vi "Detector_Controller_status_extract.vi"(10 "Status Headers":string, 11 "Status Controllers":string="\u0000Status of FitsHeader\n---------------------------------------------------------\r\nHeader0\r\nModify  : 20170204-171925568\r\nEXPTIMES: 1000\r\nEXPTIMEL: 1000\r\nNFRAMES : 1\r\nNGROUPS : 1\r\nOffsets : NOT loaded deu to write protection.\r\n          0x369 0x361 0x361 0x363 0x35a 0x357 0x360 0x361\r\n          0x34a 0x34c 0x347 0x349 0x34a 0x34b 0x349 0x349\r\n          0x351 0x350 0x353 0x351 0x351 0x351 0x350 0x353\r\n          0x350 0x352 0x353 0x352 0x353 0x351 0x351 0x355\r\n---------------------------------------------------------\r\nHeader1\r\nModify  : 20170204-171925571\r\nEXPTIMES: 2000\r\nEXPTIMEL: 1000\r\nNFRAMES : 1\r\nNGROUPS : 1\r\nOffsets : NOT loaded deu to write protection.\r\n          0x387 0x389 0x38a 0x389 0x388 0x38a 0x388 0x387\r\n          0x39c 0x39b 0x39d 0x39b 0x39d 0x39b 0x39c 0x39c\r\n          0x38f 0x38f 0x391 0x391 0x390 0x38e 0x38e 0x38e\r\n          0x38f 0x391 0x38e 0x390 0x38e 0x390 0x38f 0x38e\r\n---------------------------------------------------------") -> (2 "Params Det 1":i32[](array[numeric]), 3 "Params":i32[](array[numeric]))   [LabVIEW 2024]
uses:
  <vilib>/regexp/Match Regular Expression.xnode
panel:
  out "Controller status lines 2":string[](array[string])
  out "match + rest of string 4":string
  out "Status 2":bool[](array[boolean])
  out "Status":bool[](array[boolean])
  out "Controller status lines":string[](array[string])
  out "match + rest of string 3":string
  out "Satus of Detectors 1":string[](array[string])
  out "match + rest of string 2":string
  out "substring before match":string
  out "Array 2":i32[](array[numeric])
  out "Satus of Detector 0":string[](array[string])
  out "match + rest of string":string
  out "spreadsheet string":string
  out "after match":string
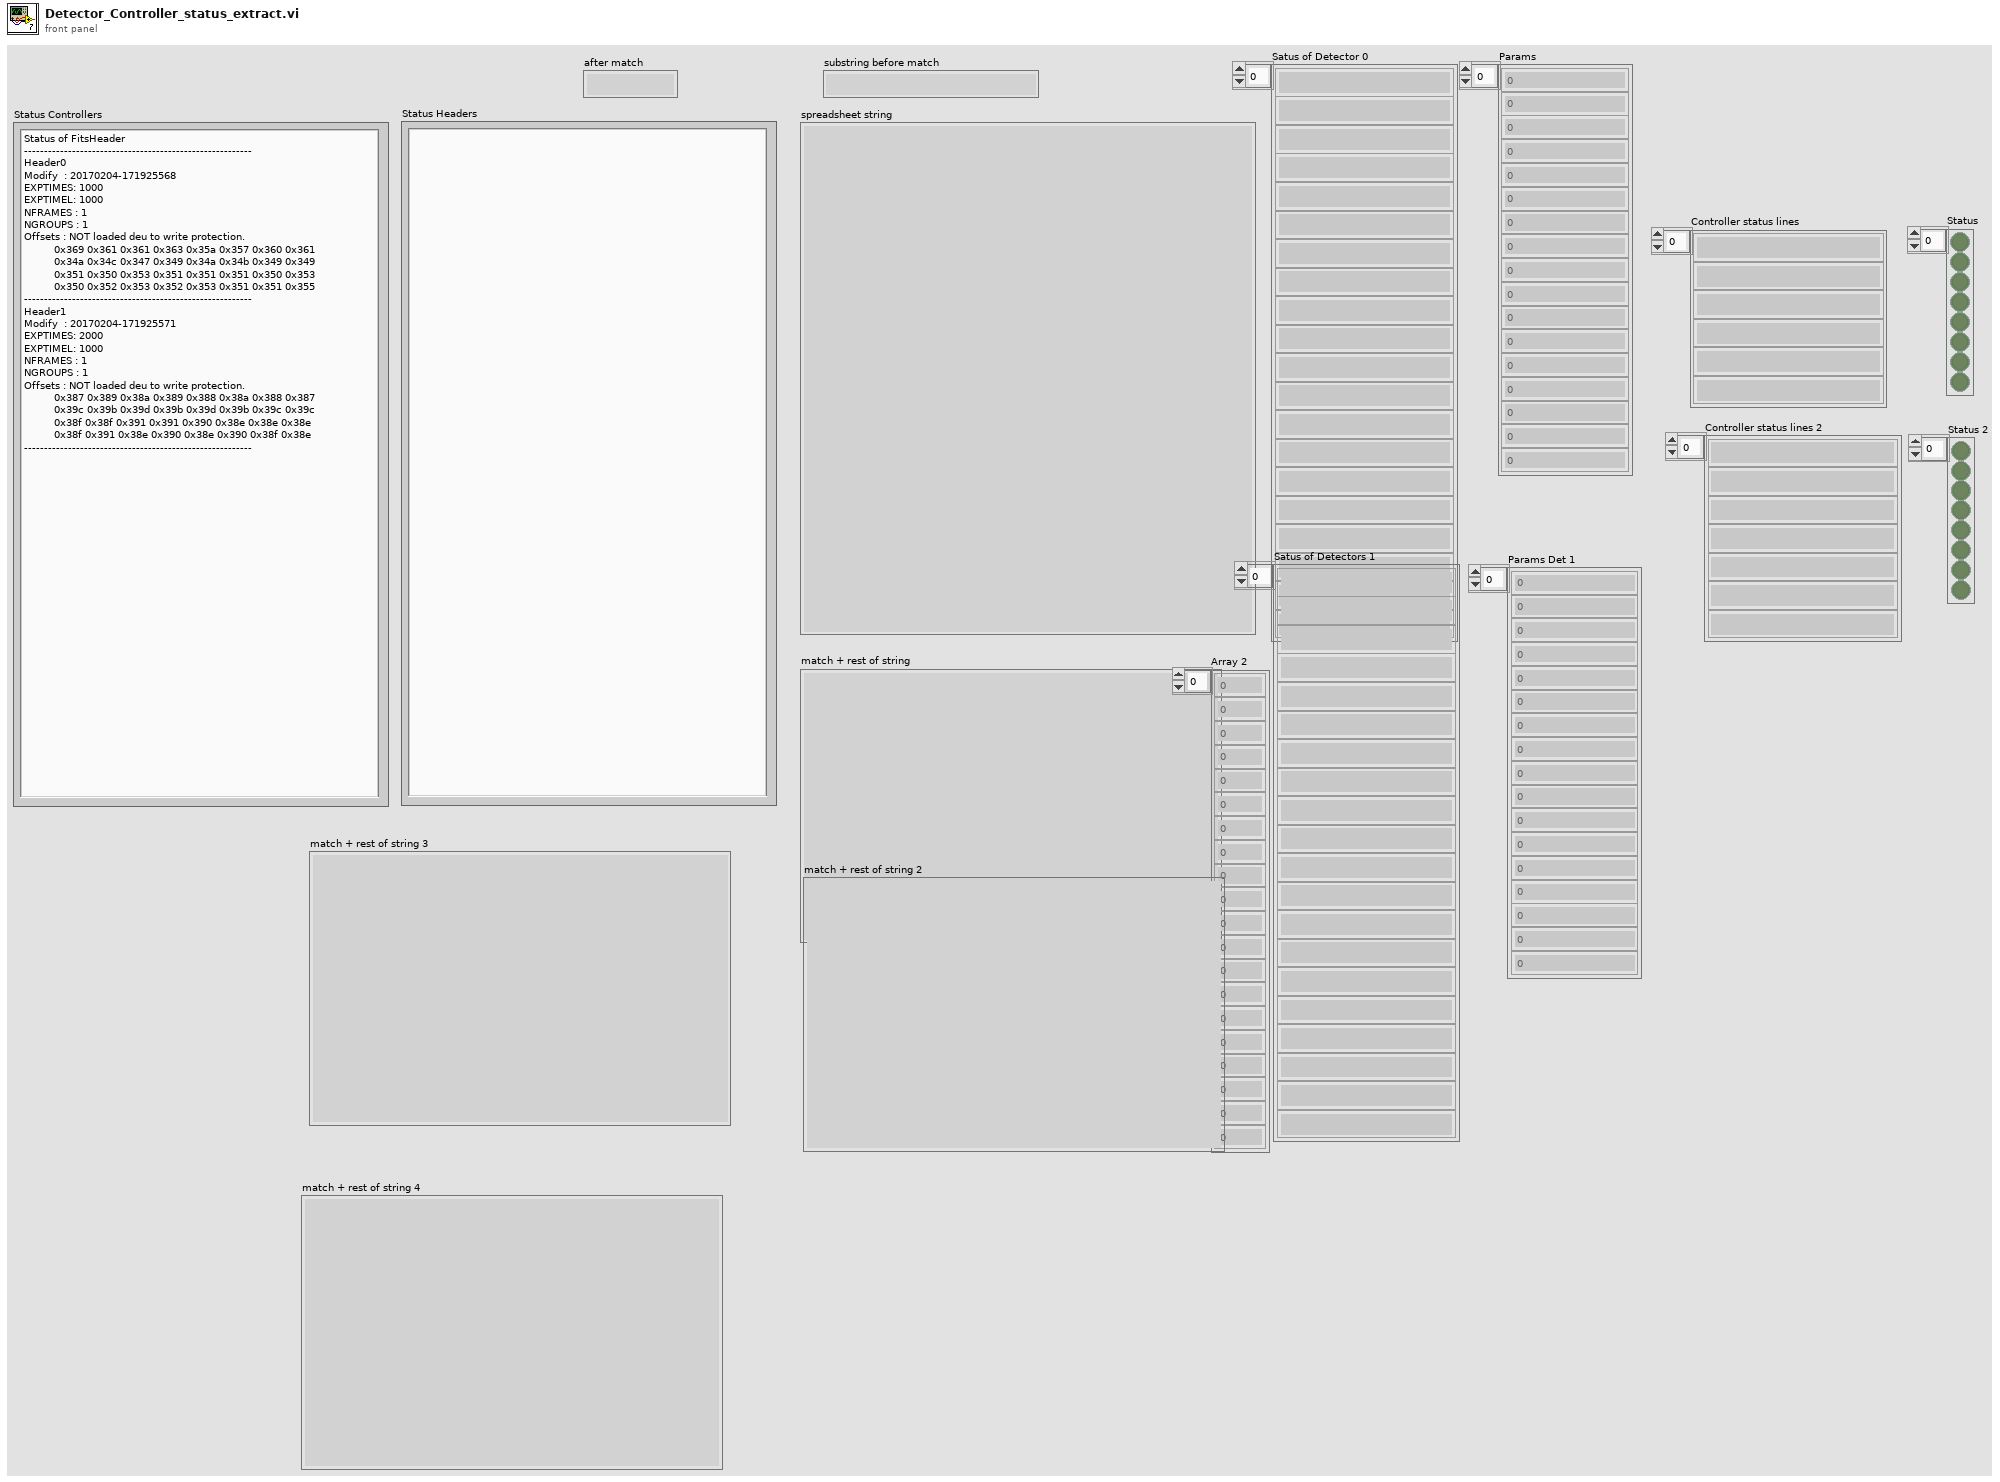
[diagram p1: front panel]
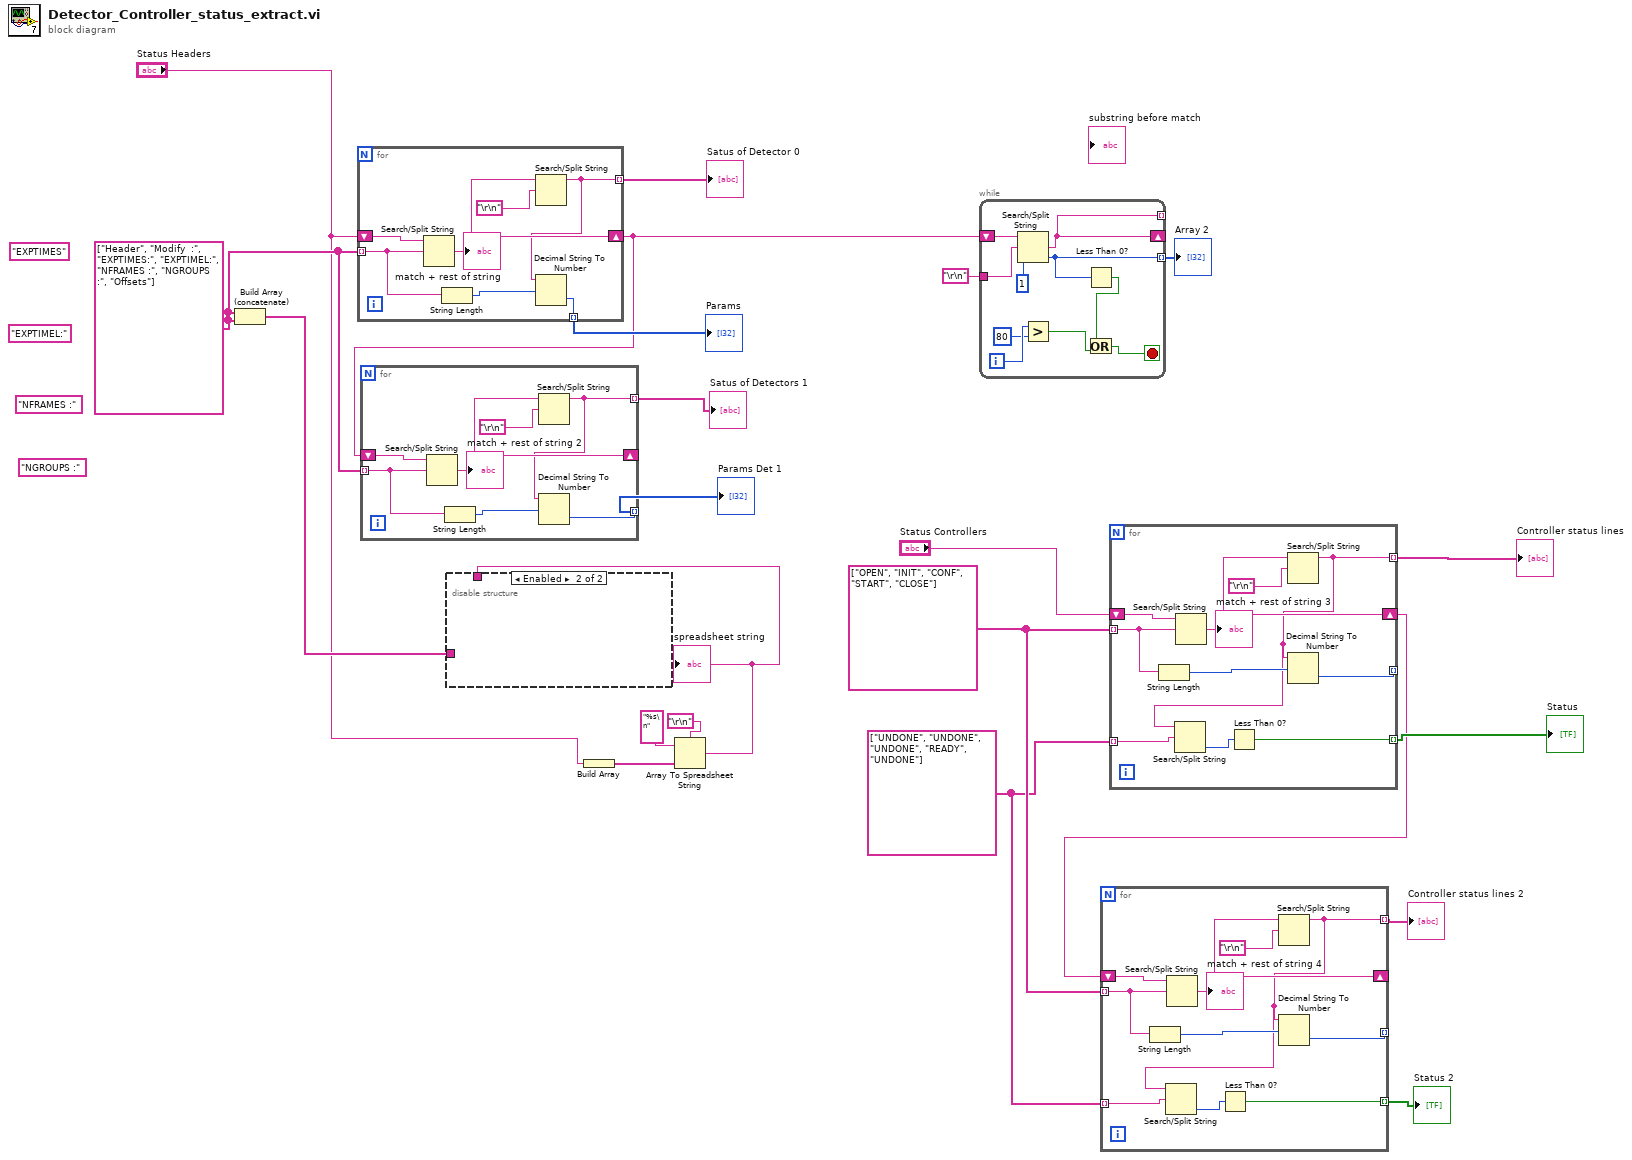
[diagram p0: block diagram]
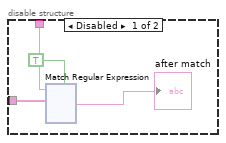
[diagram p2: hidden frame]
diagram:
  w3 = string[] ["UNDONE", "UNDONE", "UNDONE", "READY", "UNDONE"]
  w4 = string[] ["OPEN", "INIT", "CONF", "START", "CLOSE"]
  w12 = string[] ["Header", "Modify  :", "EXPTIMES:", "EXPTIMEL:", "NFRAMES :", "NGROUPS :", "Offsets"]
  (unwired) "NGROUPS :" ("Status Controllers")
  (unwired) "NFRAMES :" ("Status Controllers")
  (unwired) "EXPTIMEL:" ("Status Controllers")
  (unwired) "EXPTIMES" ("Status Controllers")
  n1 = Build Array (concatenate)(w12, w12) -> (w15:string[])
  n2 = for {
    tunnel: w12 -> [w24] mode=indexing
    tunnel: [w26] -> w16 mode=indexing
    shift-right: [w28] -> w13
    shift-left: "Status Headers" -> [w29]
    tunnel: [w25] -> w14 mode=indexing
    n3 = Search/Split String(string=w29, search string/char (-)=w24) -> (match + rest of string=w28:string)  [unwired: 1 in, 2 out]
    "match + rest of string" <- w28
    n4 = String Length(string=w24) -> (length=w23:i32)
    n5 = Search/Split String(string=w28, search string/char (-)="\r\n") -> (substring before match=w26:string)  [unwired: 1 in, 2 out]
    n6 = Decimal String To Number(string=w26, offset=w23) -> (number=w25:i32)  [unwired: 1 in, 1 out]
  }
  "Satus of Detector 0" <- w16
  "Params" <- w14
  n7 = for {
    tunnel: w12 -> [w31] mode=indexing
    tunnel: [w33] -> w11 mode=indexing
    shift-right: [w35] -> _
    shift-left: w13 -> [w36]
    tunnel: [w32] -> w10 mode=indexing
    n8 = Search/Split String(string=w36, search string/char (-)=w31) -> (match + rest of string=w35:string)  [unwired: 1 in, 2 out]
    "match + rest of string 2" <- w35
    n9 = String Length(string=w31) -> (length=w30:i32)
    n10 = Search/Split String(string=w35, search string/char (-)="\r\n") -> (substring before match=w33:string)  [unwired: 1 in, 2 out]
    n11 = Decimal String To Number(string=w33, offset=w30) -> (number=w32:i32)  [unwired: 1 in, 1 out]
  }
  "Satus of Detectors 1" <- w11
  "Params Det 1" <- w10
  n12 = Build Array("Status Headers") -> (w20:string[])
  n13 = Array To Spreadsheet String(delimiter (Tab)="\r\n", array=w20, 3:"%s\n" ("format string")) -> (spreadsheet string=w19:string)
  "spreadsheet string" <- w19
  n14 = disable-structure shown="Enabled" {
    disable-tunnel: w15 -> [w40 _]
    disable-tunnel: w19 -> [w39 _]
    frame Disabled {
      n15 = xnode "Match Regular Expression"("input string"=w39, "regular expression"=w40, "multiline? (F)"=TRUE) -> ("after match"=→"after match":string)  [unwired: 3 in, 4 out]
    }
    frame Enabled {
    }
  }
  n16 = while {
    tunnel: "\r\n" -> [w166]
    shift-right: [w158] -> _
    shift-left: w13 -> [w167]
    tunnel: [w164] -> w17 mode=indexing
    tunnel: [w158] -> _ mode=indexing
    i -> [w163]
    stop <- w159 stop-if-true
    n17 = Search/Split String(string=w167, search string/char (-)=w166, offset (0)=1) -> (match + rest of string=w158:string, offset of match=w164:i32)  [unwired: 1 out]
    n18 = Greater?(x=w163, y=80) -> (0:w161:bool)
    n19 = Less Than 0?(x=w164) -> (x < 0?=w160:bool)
    n20 = Or(x=w160, y=w161) -> (x .or. y?=w159:bool)
  }
  "Array 2" <- w17
  n21 = for {
    tunnel: w4 -> [w173] mode=indexing
    tunnel: [w170] -> w7 mode=indexing
    shift-right: [w176] -> w5
    shift-left: "Status Controllers" -> [w177]
    tunnel: [w174] -> _ mode=indexing
    tunnel: w3 -> [w171] mode=indexing
    tunnel: [w168] -> w6 mode=indexing
    n22 = String Length(string=w173) -> (length=w172:i32)
    n23 = Search/Split String(string=w177, search string/char (-)=w173) -> (match + rest of string=w176:string)  [unwired: 1 in, 2 out]
    "match + rest of string 3" <- w176
    n24 = Search/Split String(string=w176, search string/char (-)="\r\n") -> (substring before match=w170:string)  [unwired: 1 in, 2 out]
    n25 = Search/Split String(string=w170, search string/char (-)=w171) -> (offset of match=w169:i32)  [unwired: 1 in, 2 out]
    n26 = Less Than 0?(x=w169) -> (x < 0?=w168:bool)
    n27 = Decimal String To Number(string=w170, offset=w172) -> (number=w174:i32)  [unwired: 1 in, 1 out]
  }
  "Controller status lines" <- w7
  "Status" <- w6
  n28 = for {
    tunnel: w4 -> [w183] mode=indexing
    tunnel: [w180] -> w1 mode=indexing
    shift-right: [w186] -> _
    shift-left: w5 -> [w187]
    tunnel: [w184] -> _ mode=indexing
    tunnel: w3 -> [w181] mode=indexing
    tunnel: [w178] -> w2 mode=indexing
    n29 = String Length(string=w183) -> (length=w182:i32)
    n30 = Search/Split String(string=w187, search string/char (-)=w183) -> (match + rest of string=w186:string)  [unwired: 1 in, 2 out]
    "match + rest of string 4" <- w186
    n31 = Search/Split String(string=w186, search string/char (-)="\r\n") -> (substring before match=w180:string)  [unwired: 1 in, 2 out]
    n32 = Search/Split String(string=w180, search string/char (-)=w181) -> (offset of match=w179:i32)  [unwired: 1 in, 2 out]
    n33 = Less Than 0?(x=w179) -> (x < 0?=w178:bool)
    n34 = Decimal String To Number(string=w180, offset=w182) -> (number=w184:i32)  [unwired: 1 in, 1 out]
  }
  "Status 2" <- w2
  "Controller status lines 2" <- w1
